vi "in1.vi"() -> ()   [LabVIEW 2018]
panel:
  out "Waveform Graph":dynamicdata(graph)
  in  "stop (F)":bool
  in  "timeout (s)":dbl=30.0 format="%0.2f"
  in  "number of samples":i32=100
  in  "rate":dbl=10000.0
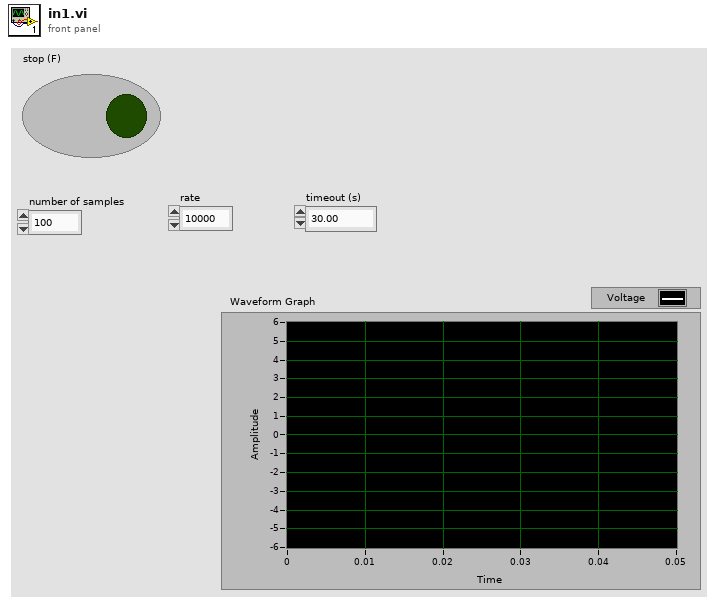
[diagram p1: front panel]
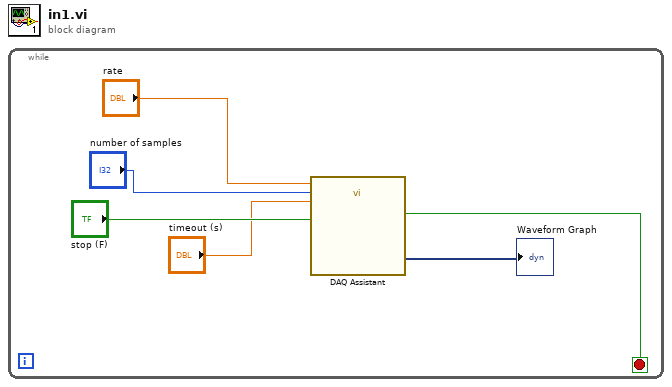
[diagram p0: block diagram]
diagram:
  n1 = while {
    stop <- w5 stop-if-true
    n2 = call "DAQ Assistant"("rate"="rate", "number of samples"="number of samples", "timeout (s)"="timeout (s)", "stop (F)"="stop (F)") -> ("data"=→"Waveform Graph":dynamicdata, "stopped"=w5:bool)  [unwired: 12 in, 2 out]
  }
